vi "BSC203 multichannel control - basic.vi"() -> ()   [LabVIEW 2011]
uses:
  C:/Users/nbayconich/Documents/Kinesis APT motion control programming/Kinesis labview project Nick test/Thorlabs.MotionControl.Controls.dll
  Thorlabs.MotionControl.Controls.dll
  C:/Users/nbayconich/Documents/Kinesis APT motion control programming/Kinesis labview project Nick test/Thorlabs.MotionControl.Benchtop.StepperMotorCLI.dll
  Thorlabs.MotionControl.Benchtop.StepperMotorCLI.dll
  C:/Users/nbayconich/Documents/Kinesis APT motion control programming/Kinesis labview project Nick test/Thorlabs.MotionControl.GenericMotorCLI.dll
  Thorlabs.MotionControl.GenericMotorCLI.dll
panel:
  out "Initialization\nError":errorcluster
  out "Channel 3\nEnabled?":bool
  out "Channel 2 \nEnabled?":bool
  out "Channel 1\nEnabled?":bool
  in  "Stop Control":bool
  in  "Controller Serial Number":string="70XXXXXX"
  in  "Benchtop Stepper Controller 3":refnum<k24>(container)
  in  "Benchtop Stepper Controller 2":refnum<k24>(container)
  in  "Benchtop Stepper Controller":refnum<k24>(container)
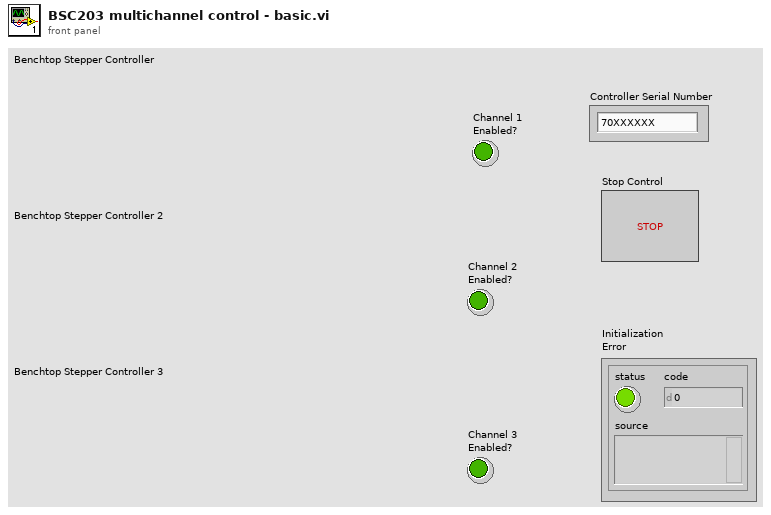
[diagram p1: front panel]
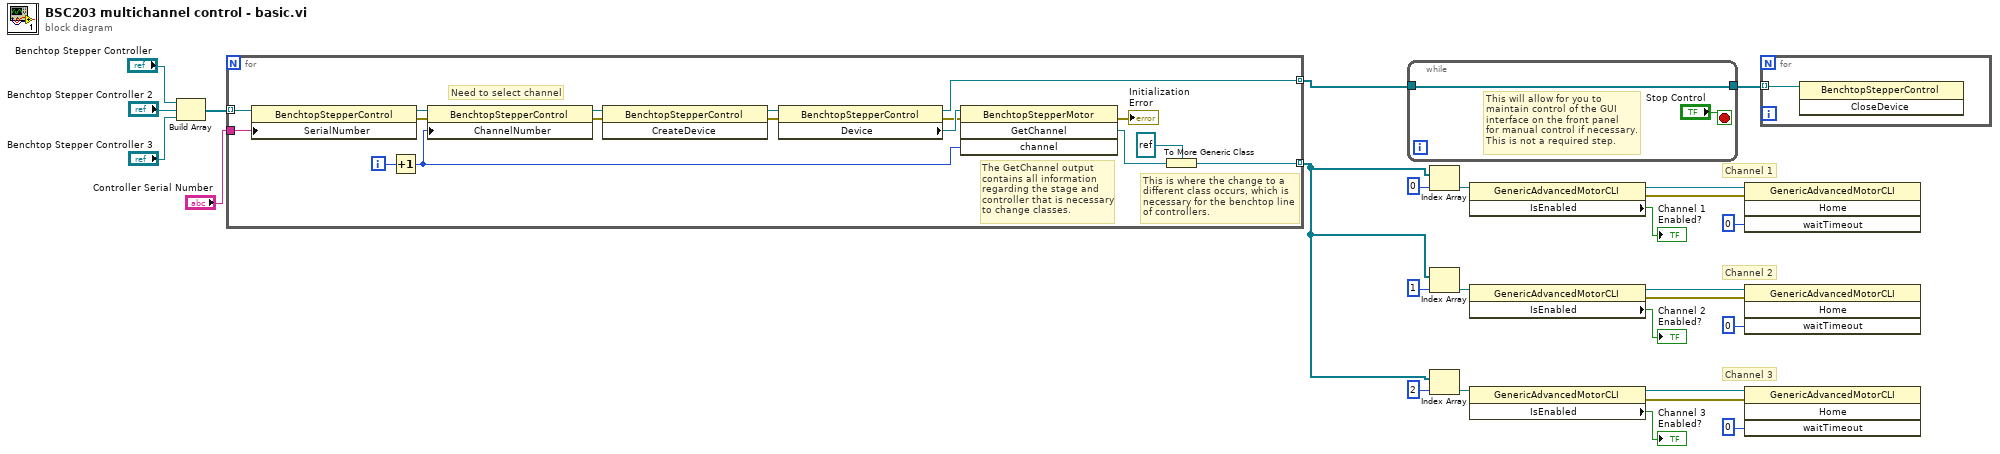
[diagram p0: block diagram]
diagram:
  # "Channel 3"
  # "Channel 2"
  # "Channel 1"
  n1 = Build Array("Benchtop Stepper Controller", "Benchtop Stepper Controller 2", "Benchtop Stepper Controller 3") -> (w23:refnum<k24>[])
  n2 = for {
    tunnel: w23 -> [w43] mode=indexing
    tunnel: "Controller Serial Number" -> [w42]
    tunnel: [w33] -> w17 mode=indexing
    tunnel: [w28] -> w21 mode=indexing
    i -> [w37]
    # "This is where the change to a\ndifferent class occurs, which is \nnecessary for the benchtop line\nof controllers."
    # "The GetChannel output\ncontains all information\nregarding the stage and\ncontroller that is necessary\nto change classes."
    # "Need to select channel"
    n3 = property class="BenchtopStepperControl"(reference=w43, "SerialNumber"=w42) -> (reference out=w39:refnum<k24>, error out=w38:errorcluster)  [unwired: 1 in]
    n4 = Increment(x=w37) -> (x+1=w32:i32)
    n5 = property class="BenchtopStepperControl"(reference=w39, error in=w38, "ChannelNumber"=w32) -> (reference out=w35:refnum<k24>, error out=w36:errorcluster)
    n6 = invoke class="BenchtopStepperControl" method="CreateDevice"(reference=w35, error in=w36) -> (reference out=w41:refnum<k24>, error out=w40:errorcluster)  [unwired: 1 in, 1 out]
    n7 = property class="BenchtopStepperControl"(reference=w41, error in=w40) -> (reference out=w33:refnum<k24>, error out=w31:errorcluster, "Device"=w34:refnum<k24>)
    n8 = invoke class="BenchtopStepperMotor" method="GetChannel"(reference=w34, error in=w31, "channel"=w32) -> (error out=→"Initialization\nError":errorcluster, "GetChannel"=w30:refnum<k24>)  [unwired: 1 in, 2 out]
    n9 = To More Generic Class(target class=refnum<k24> refnum, reference=w30) -> (generic class reference=w28:refnum<k24>)
  }
  n10 = while {
    tunnel: [w44] -> w16
    tunnel: w17 -> [w44]
    stop <- "Stop Control" stop-if-true
    # "This will allow for you to\nmaintain control of the GUI\ninterface on the front panel\nfor manual control if necessary.\nThis is not a required step."
  }
  n11 = Index Array(array=w21, index=0) -> (element=w12:refnum<k24>)
  n12 = Index Array(array=w21, index=1) -> (element=w6:refnum<k24>)
  n13 = Index Array(array=w21, index=2) -> (element=w7:refnum<k24>)
  n14 = property class="GenericAdvancedMotorCLI"(reference=w12) -> (reference out=w8:refnum<k24>, error out=w2:errorcluster, "IsEnabled"=→"Channel 1\nEnabled?":bool)  [unwired: 1 in]
  n15 = property class="GenericAdvancedMotorCLI"(reference=w6) -> (reference out=w5:refnum<k24>, error out=w3:errorcluster, "IsEnabled"=→"Channel 2 \nEnabled?":bool)  [unwired: 1 in]
  n16 = property class="GenericAdvancedMotorCLI"(reference=w7) -> (reference out=w4:refnum<k24>, error out=w1:errorcluster, "IsEnabled"=→"Channel 3\nEnabled?":bool)  [unwired: 1 in]
  n17 = invoke class="GenericAdvancedMotorCLI" method="Home"(reference=w8, error in=w2, "waitTimeout"=0) -> ()  [unwired: 1 in, 4 out]
  n18 = invoke class="GenericAdvancedMotorCLI" method="Home"(reference=w5, error in=w3, "waitTimeout"=0) -> ()  [unwired: 1 in, 4 out]
  n19 = invoke class="GenericAdvancedMotorCLI" method="Home"(reference=w4, error in=w1, "waitTimeout"=0) -> ()  [unwired: 1 in, 4 out]
  n20 = for {
    tunnel: w16 -> [w46] mode=indexing
    n21 = invoke class="BenchtopStepperControl" method="CloseDevice"(reference=w46) -> ()  [unwired: 2 in, 3 out]
  }
